vi "Launch Nested Actors.vi"(8 "error in (no error)":errorcluster, 11 "Elevator Controller Actor in":refnum<class "Elevator Controller Actor.lvclass">) -> (0 "error out":errorcluster, 3 "Elevator Controller Actor out":refnum<class "Elevator Controller Actor.lvclass">)   [LabVIEW 2019, in "Elevator Controller Actor.lvlib" / "Elevator Controller Actor.lvclass"]
uses:
  Elevator Controller Actor.lvclass
  <vilib>/ActorFramework/Actor/Actor.lvclass
  Sim User Console Actor/Elevator Controller/Sim User Console Actor.lvclass
  Sim Display Console Actor/Elevator Controller/Sim Display Console Actor.lvclass
  Simulated Sensor Interface Actor/Elevator Controller/Sim Sensor Interface.lvclass
  Configuration Database Actor/Configuration Database Actor/Configuration Database Actor.lvclass
  C:/Program Files (x86)/National Instruments/LabVIEW 2019/vi.lib/ActorFramework/Actor/Actor.lvclass
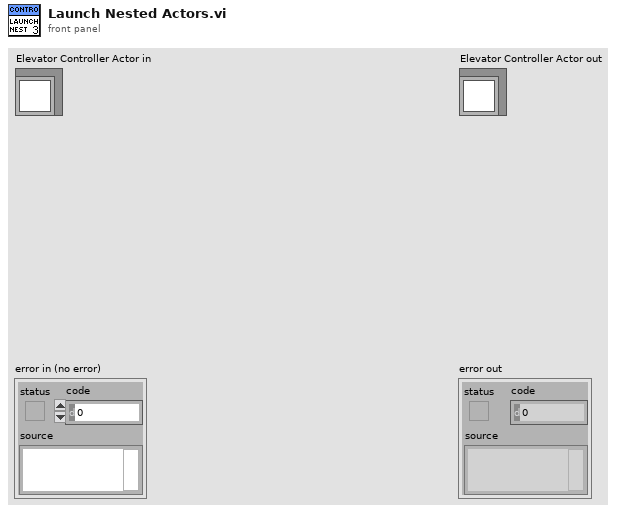
[diagram p1: front panel]
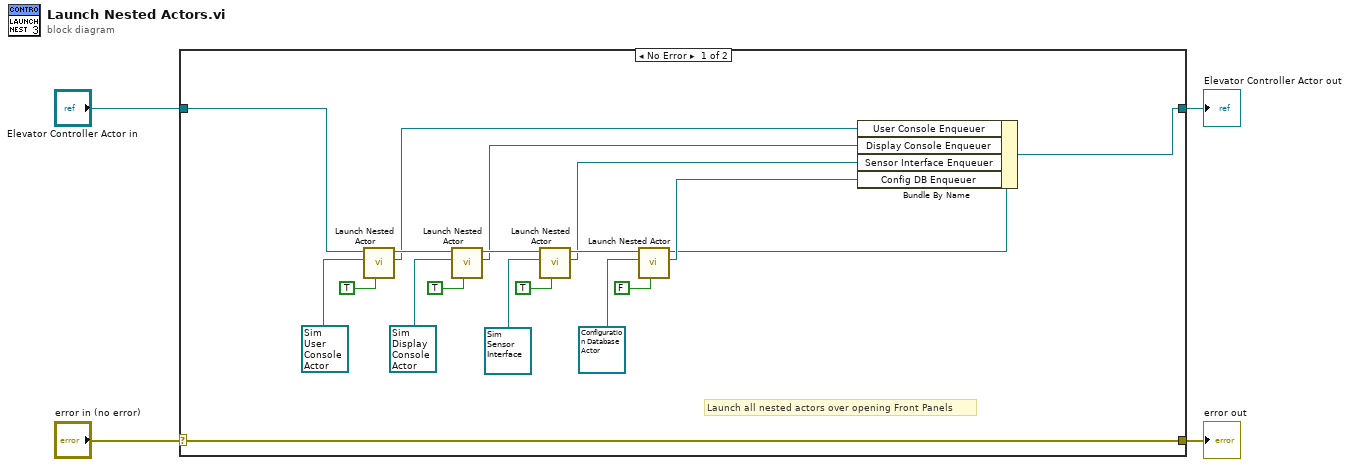
[diagram p0: block diagram]
diagram:
  n1 = case shown="No Error" "error in (no error)" {
    selector: "error in (no error)" -> [w23 w25]
    tunnel: [w23 w25] -> w3
    tunnel: [w14 w24] -> w1
    tunnel: "Elevator Controller Actor in" -> [w15 w24]
    frame No Error {
      # "Launch all nested actors over opening Front Panels"
      n2 = call <vilib>:"Launch Nested Actor.vi"("Open Actor Core front panel? (F)"=TRUE, "Nested Actor"=refnum<class "Sim User Console Actor.lvclass"> refnum ("Simulated User Console Actor.lvlib:Sim User Console Actor.lvclass"), "Caller Actor in"=w15) -> ("Nested Actor's Enqueuer"=w13:refnum<class "Message Enqueuer.lvclass">, "Caller Actor out"=w22:refnum<class "Elevator Controller Actor.lvclass">)  [unwired: 6 in, 1 out]
      n3 = call <vilib>:"Launch Nested Actor.vi"("Open Actor Core front panel? (F)"=TRUE, "Nested Actor"=refnum<class "Sim Display Console Actor.lvclass"> refnum ("Simulated Display Console Actor.lvlib:Sim Display Console Actor.lvclass"), "Caller Actor in"=w22) -> ("Nested Actor's Enqueuer"=w9:refnum<class "Message Enqueuer.lvclass">, "Caller Actor out"=w21:refnum<class "Elevator Controller Actor.lvclass">)  [unwired: 6 in, 1 out]
      n4 = call <vilib>:"Launch Nested Actor.vi"("Open Actor Core front panel? (F)"=TRUE, "Nested Actor"=refnum<class "Sim Sensor Interface.lvclass"> refnum ("Simulated Sensor Interface Actor.lvlib:Sim Sensor Interface.lvclass"), "Caller Actor in"=w21) -> ("Nested Actor's Enqueuer"=w7:refnum<class "Message Enqueuer.lvclass">, "Caller Actor out"=w20:refnum<class "Elevator Controller Actor.lvclass">)  [unwired: 6 in, 1 out]
      n5 = call <vilib>:"Launch Nested Actor.vi"("Open Actor Core front panel? (F)"=FALSE, "Nested Actor"=refnum<class "Configuration Database Actor.lvclass"> refnum ("Configuration Database Actor.lvlib:Configuration Database Actor.lvclass"), "Caller Actor in"=w20) -> ("Nested Actor's Enqueuer"=w6:refnum<class "Message Enqueuer.lvclass">, "Caller Actor out"=w5:refnum<class "Elevator Controller Actor.lvclass">)  [unwired: 6 in, 1 out]
      n6 = Bundle By Name(cluster=w5, "User Console Enqueuer"=w13, "Display Console Enqueuer"=w9, "Sensor Interface Enqueuer"=w7, "Config DB Enqueuer"=w6) -> (w14:refnum<class "Elevator Controller Actor.lvclass">)
    }
    frame Error {
    }
  }
  "error out" <- w3
  "Elevator Controller Actor out" <- w1
